vi "RTS Plot TCP Data.vi"(0 "Chamber 1 Socket":string[][](array[string]), 1 "Chamber 2 Socket":string[][](array[string]), 2 "Chamber 3 Socket":string[][](array[string]), 3 "Chamber 4 Socket":string[][](array[string]), 4 "Tree Selection in":T2, 5 "Error In":errorcluster, 9 "CSV Data in":T1 {"Station 1" format="%.6f"; "Station 2" format="%.6f"; "Station 3" format="%.6f"; "Station 4" format="%.6f"; "Station 5" format="%.6f"; "Station 6" format="%.6f"; "Station 7" format="%.6f"; "Station 8" format="%.6f"}) -> (10 "Chamber Data":string[][](array[string]), 13 "Full Item Names":string[](array[string]), 14 "Point File Name":string, 15 "CSV Data out":T1 {"Station 1" format="%.6f"; "Station 2" format="%.6f"; "Station 3" format="%.6f"; "Station 4" format="%.6f"; "Station 5" format="%.6f"; "Station 6" format="%.6f"; "Station 7" format="%.6f"; "Station 8" format="%.6f"}, 16 "Custom Titles":string[](array[string]), 17 "Listbox Data":string[][](array[string]), 18 "Tree Selection out":T2="Select Room/Stall", 19 "Error Out":errorcluster)   [LabVIEW 2020]
uses:
  Type Definitions/RTS TDMS Data.ctl
  Type Definitions/RTS Room Selector.ctl
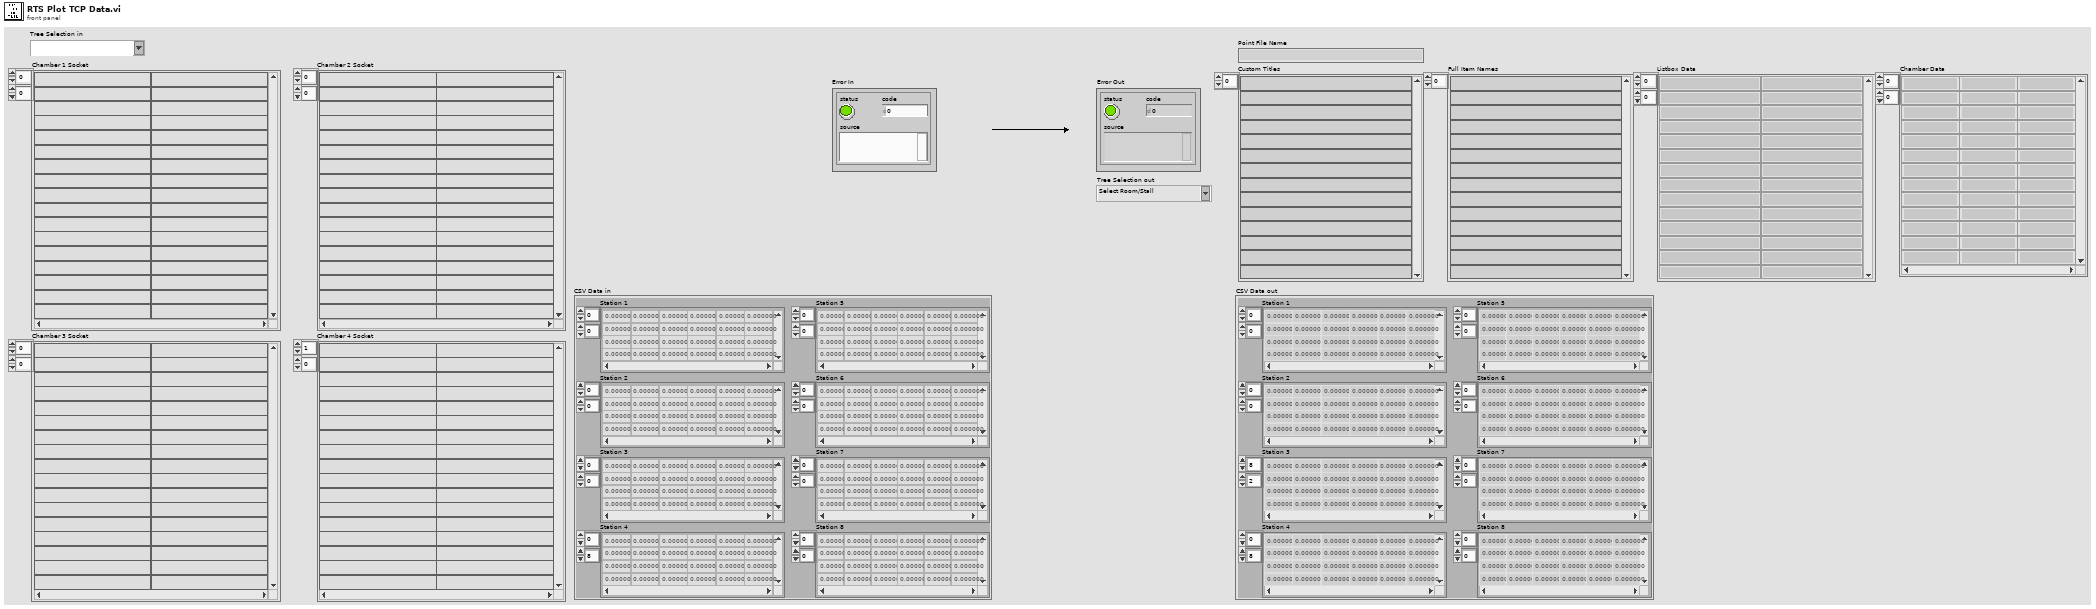
[diagram p1: front panel]
types:
  T1 = typedef "RTS TDMS Data.ctl" = cluster{"Station 1":dbl[][], "Station 2":dbl[][], "Station 3":dbl[][], "Station 4":dbl[][], "Station 5":dbl[][], "Station 6":dbl[][], "Station 7":dbl[][], "Station 8":dbl[][]}
  T2 = typedef "RTS Room Selector.ctl" = string
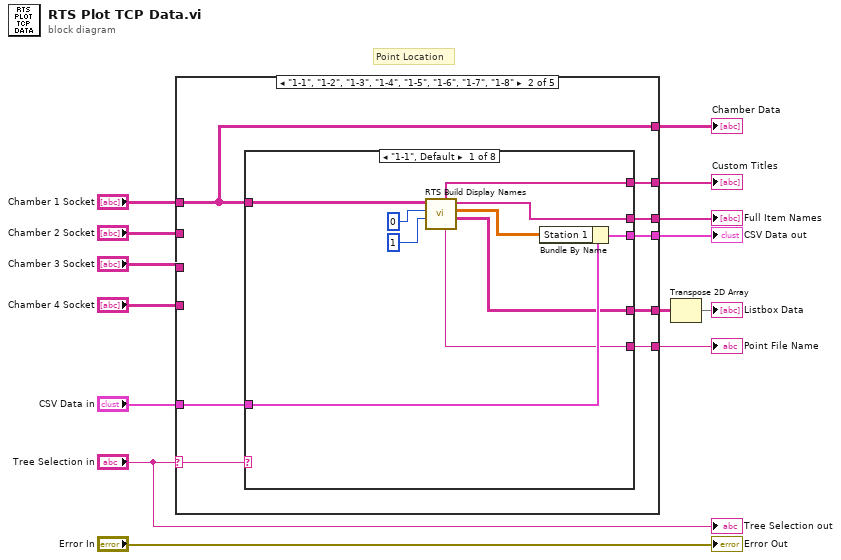
[diagram p0: block diagram]
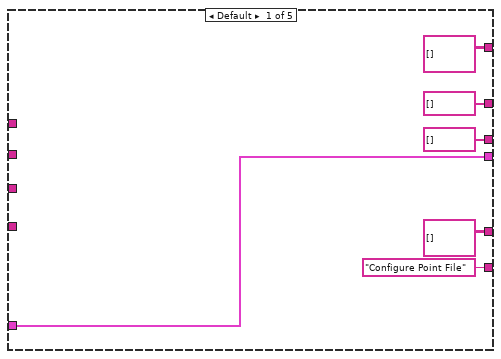
[diagram p2: hidden frame]
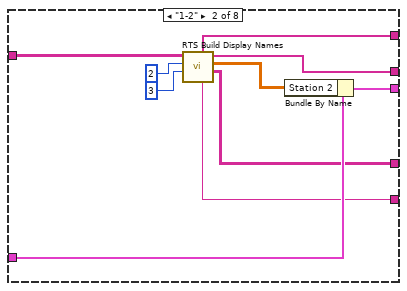
[diagram p3: hidden frame]
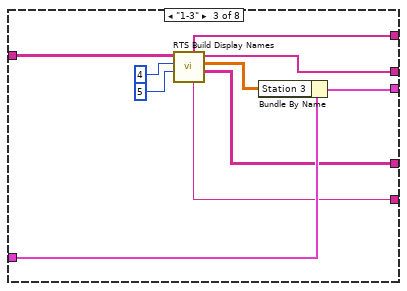
[diagram p4: hidden frame]
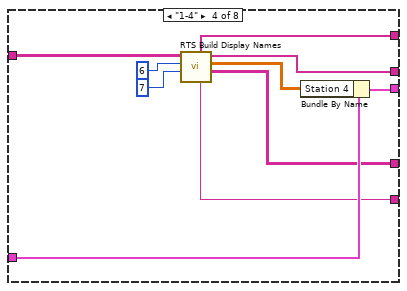
[diagram p5: hidden frame]
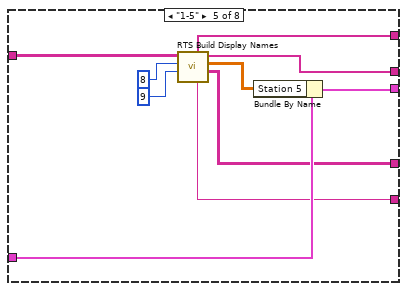
[diagram p6: hidden frame]
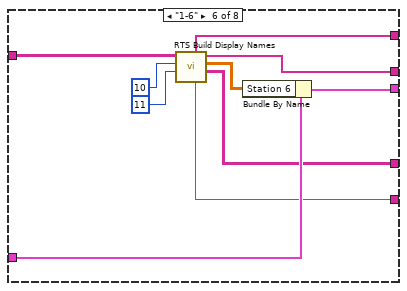
[diagram p7: hidden frame]
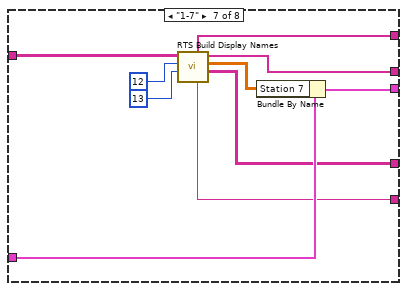
[diagram p8: hidden frame]
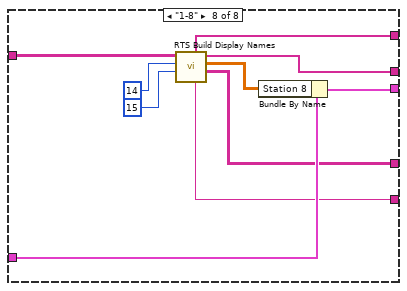
[diagram p9: hidden frame]
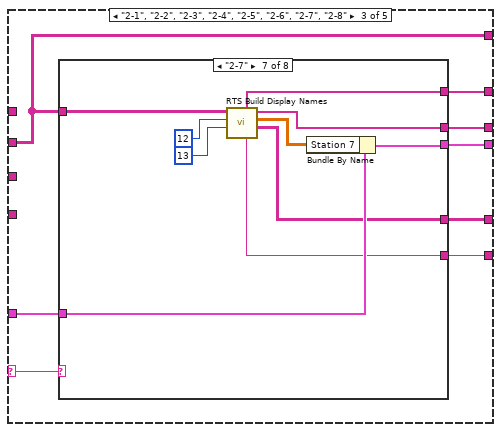
[diagram p10: hidden frame]
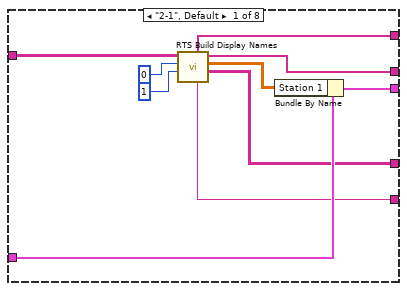
[diagram p11: hidden frame]
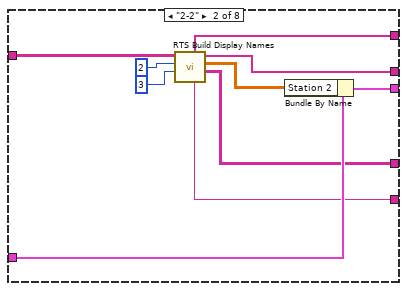
[diagram p12: hidden frame]
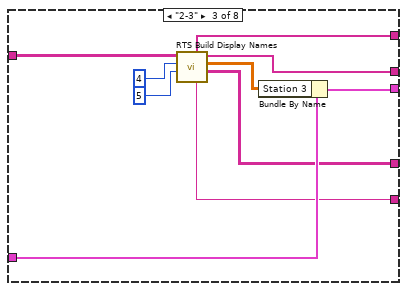
[diagram p13: hidden frame]
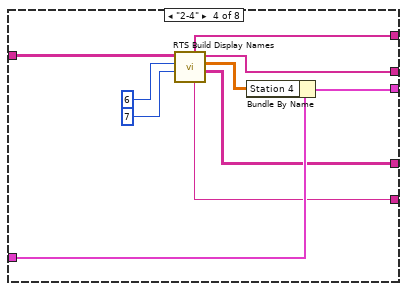
[diagram p14: hidden frame]
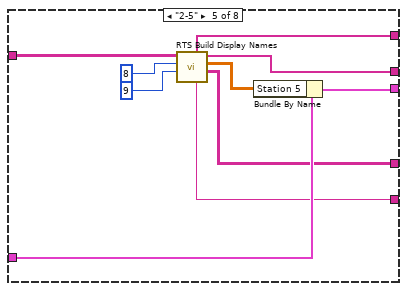
[diagram p15: hidden frame]
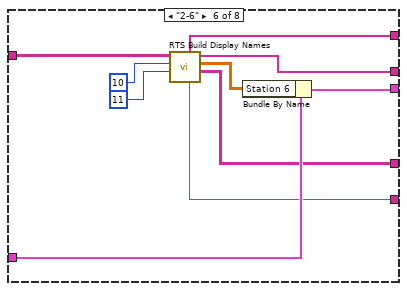
[diagram p16: hidden frame]
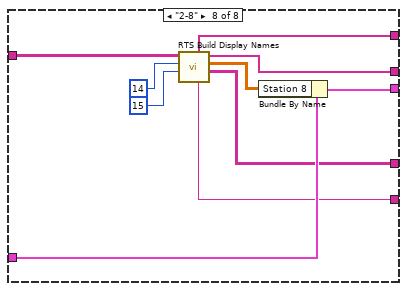
[diagram p17: hidden frame]
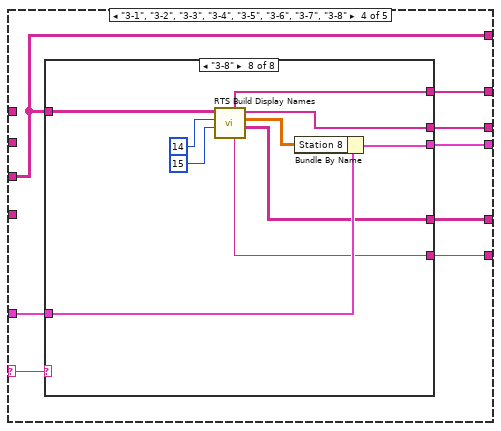
[diagram p18: hidden frame]
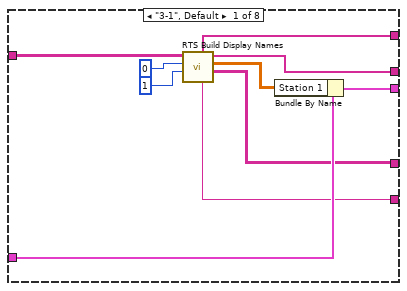
[diagram p19: hidden frame]
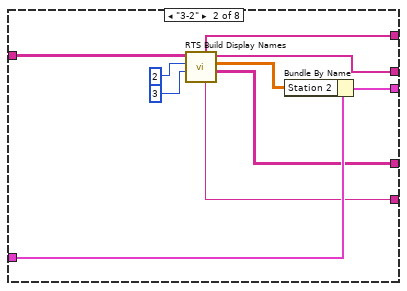
[diagram p20: hidden frame]
diagram:
  # "Point Location"
  n1 = case shown="\"1-1\", \"1-2\", \"1-3\", \"1-4\", \"1-5\", \"1-6\", \"1-7\", \"1-8\"" "Tree Selection in" {
    selector: "Tree Selection in" -> [_ w25 w113 w203 w291]
    tunnel: "Chamber 1 Socket" -> [_ w23 _ _ _]
    tunnel: "Chamber 2 Socket" -> [_ _ w111 _ _]
    tunnel: "Chamber 3 Socket" -> [_ _ _ w199 _]
    tunnel: "Chamber 4 Socket" -> [_ _ _ _ w287]
    tunnel: [string[] [] ("Chamber 4 Socket") w28 w114 w202 w290] -> w14
    tunnel: "CSV Data in" -> [w19 w27 w116 w204 w292]
    tunnel: [w19 w26 w115 w201 w289] -> w12
    tunnel: [string[][] [] w24 w112 w200 w288] -> w5
    tunnel: [string[][] [] ("Chamber 4 Socket") w23 w111 w199 w287] -> w3
    tunnel: [string[] [] ("Custom Titles") w22 w110 w198 w286] -> w2
    tunnel: ["Configure Point File" ("Point File Name") w21 w109 w197 w285] -> w1
    frame Default {
    }
    frame "1-1", "1-2", "1-3", "1-4", "1-5", "1-6", "1-7", "1-8" {
      n2 = case shown="\"1-1\", Default" w25 {
        tunnel: w23 -> [w38 w46 w56 w66 w76 w86 w96 w106]
        tunnel: [w32 w45 w53 w65 w75 w85 w95 w105] -> w28
        tunnel: w27 -> [w35 w48 w58 w68 w78 w88 w98 w108]
        tunnel: [w33 w47 w57 w67 w77 w87 w97 w107] -> w26
        tunnel: [w31 w43 w51 w63 w73 w83 w91 w103] -> w24
        tunnel: [w30 w40 w50 w60 w70 w80 w90 w100] -> w22
        tunnel: [w29 w39 w49 w59 w69 w79 w89 w99] -> w21
        frame "1-1", Default {
          n3 = call "RTS Build Display Names.vi"("Data Row"=1 ("index (row)"), "Name Row"=0 ("index (row)"), "Chamber 1 Socket in"=w38) -> ("Listbox Data"=w31:string[][], "DBL Plot Data"=w34:dbl[][], "Full Item Names"=w32:string[], "Point File Name"=w29:string, "Custom Titles"=w30:string[])  [unwired: 4 in]
          n4 = Bundle By Name(cluster=w35, "Station 1"=w34) -> (w33:T1)
        }
        frame "1-2" {
          n5 = call "RTS Build Display Names.vi"("Data Row"=3 ("index (row)"), "Name Row"=2 ("index (row)"), "Chamber 1 Socket in"=w46) -> ("Listbox Data"=w43:string[][], "DBL Plot Data"=w44:dbl[][], "Full Item Names"=w45:string[], "Point File Name"=w39:string, "Custom Titles"=w40:string[])  [unwired: 4 in]
          n6 = Bundle By Name(cluster=w48, "Station 2"=w44) -> (w47:T1)
        }
        frame "1-3" {
          n7 = call "RTS Build Display Names.vi"("Data Row"=5 ("index (row)"), "Name Row"=4 ("index (row)"), "Chamber 1 Socket in"=w56) -> ("Listbox Data"=w51:string[][], "DBL Plot Data"=w52:dbl[][], "Full Item Names"=w53:string[], "Point File Name"=w49:string, "Custom Titles"=w50:string[])  [unwired: 4 in]
          n8 = Bundle By Name(cluster=w58, "Station 3"=w52) -> (w57:T1)
        }
        frame "1-4" {
          n9 = call "RTS Build Display Names.vi"("Data Row"=7 ("index (row)"), "Name Row"=6 ("index (row)"), "Chamber 1 Socket in"=w66) -> ("Listbox Data"=w63:string[][], "DBL Plot Data"=w64:dbl[][], "Full Item Names"=w65:string[], "Point File Name"=w59:string, "Custom Titles"=w60:string[])  [unwired: 4 in]
          n10 = Bundle By Name(cluster=w68, "Station 4"=w64) -> (w67:T1)
        }
        frame "1-5" {
          n11 = call "RTS Build Display Names.vi"("Data Row"=9 ("index (row)"), "Name Row"=8 ("index (row)"), "Chamber 1 Socket in"=w76) -> ("Listbox Data"=w73:string[][], "DBL Plot Data"=w74:dbl[][], "Full Item Names"=w75:string[], "Point File Name"=w69:string, "Custom Titles"=w70:string[])  [unwired: 4 in]
          n12 = Bundle By Name(cluster=w78, "Station 5"=w74) -> (w77:T1)
        }
        frame "1-6" {
          n13 = call "RTS Build Display Names.vi"("Data Row"=11 ("index (row)"), "Name Row"=10 ("index (row)"), "Chamber 1 Socket in"=w86) -> ("Listbox Data"=w83:string[][], "DBL Plot Data"=w84:dbl[][], "Full Item Names"=w85:string[], "Point File Name"=w79:string, "Custom Titles"=w80:string[])  [unwired: 4 in]
          n14 = Bundle By Name(cluster=w88, "Station 6"=w84) -> (w87:T1)
        }
        frame "1-7" {
          n15 = call "RTS Build Display Names.vi"("Data Row"=13 ("index (row)"), "Name Row"=12 ("index (row)"), "Chamber 1 Socket in"=w96) -> ("Listbox Data"=w91:string[][], "DBL Plot Data"=w94:dbl[][], "Full Item Names"=w95:string[], "Point File Name"=w89:string, "Custom Titles"=w90:string[])  [unwired: 4 in]
          n16 = Bundle By Name(cluster=w98, "Station 7"=w94) -> (w97:T1)
        }
        frame "1-8" {
          n17 = call "RTS Build Display Names.vi"("Data Row"=15 ("index (row)"), "Name Row"=14 ("index (row)"), "Chamber 1 Socket in"=w106) -> ("Listbox Data"=w103:string[][], "DBL Plot Data"=w104:dbl[][], "Full Item Names"=w105:string[], "Point File Name"=w99:string, "Custom Titles"=w100:string[])  [unwired: 4 in]
          n18 = Bundle By Name(cluster=w108, "Station 8"=w104) -> (w107:T1)
        }
      }
    }
    frame "2-1", "2-2", "2-3", "2-4", "2-5", "2-6", "2-7", "2-8" {
      n19 = case shown="\"2-7\"" w113 {
        tunnel: w111 -> [w124 w134 w144 w154 w164 w174 w184 w194]
        tunnel: [w123 w133 w143 w153 w163 w173 w183 w193] -> w114
        tunnel: w116 -> [w126 w136 w146 w156 w166 w176 w186 w196]
        tunnel: [w125 w135 w145 w155 w165 w175 w185 w195] -> w115
        tunnel: [w121 w131 w141 w151 w161 w171 w181 w189] -> w112
        tunnel: [w118 w128 w138 w148 w158 w168 w178 w188] -> w110
        tunnel: [w117 w127 w137 w147 w157 w167 w177 w187] -> w109
        frame "2-1", Default {
          n20 = call "RTS Build Display Names.vi"("Data Row"=1 ("index (row)"), "Name Row"=0 ("index (row)"), "Chamber 1 Socket in"=w124) -> ("Listbox Data"=w121:string[][], "DBL Plot Data"=w122:dbl[][], "Full Item Names"=w123:string[], "Point File Name"=w117:string, "Custom Titles"=w118:string[])  [unwired: 4 in]
          n21 = Bundle By Name(cluster=w126, "Station 1"=w122) -> (w125:T1)
        }
        frame "2-2" {
          n22 = call "RTS Build Display Names.vi"("Data Row"=3 ("index (row)"), "Name Row"=2 ("index (row)"), "Chamber 1 Socket in"=w134) -> ("Listbox Data"=w131:string[][], "DBL Plot Data"=w132:dbl[][], "Full Item Names"=w133:string[], "Point File Name"=w127:string, "Custom Titles"=w128:string[])  [unwired: 4 in]
          n23 = Bundle By Name(cluster=w136, "Station 2"=w132) -> (w135:T1)
        }
        frame "2-3" {
          n24 = call "RTS Build Display Names.vi"("Data Row"=5 ("index (row)"), "Name Row"=4 ("index (row)"), "Chamber 1 Socket in"=w144) -> ("Listbox Data"=w141:string[][], "DBL Plot Data"=w142:dbl[][], "Full Item Names"=w143:string[], "Point File Name"=w137:string, "Custom Titles"=w138:string[])  [unwired: 4 in]
          n25 = Bundle By Name(cluster=w146, "Station 3"=w142) -> (w145:T1)
        }
        frame "2-4" {
          n26 = call "RTS Build Display Names.vi"("Data Row"=7 ("index (row)"), "Name Row"=6 ("index (row)"), "Chamber 1 Socket in"=w154) -> ("Listbox Data"=w151:string[][], "DBL Plot Data"=w152:dbl[][], "Full Item Names"=w153:string[], "Point File Name"=w147:string, "Custom Titles"=w148:string[])  [unwired: 4 in]
          n27 = Bundle By Name(cluster=w156, "Station 4"=w152) -> (w155:T1)
        }
        frame "2-5" {
          n28 = call "RTS Build Display Names.vi"("Data Row"=9 ("index (row)"), "Name Row"=8 ("index (row)"), "Chamber 1 Socket in"=w164) -> ("Listbox Data"=w161:string[][], "DBL Plot Data"=w162:dbl[][], "Full Item Names"=w163:string[], "Point File Name"=w157:string, "Custom Titles"=w158:string[])  [unwired: 4 in]
          n29 = Bundle By Name(cluster=w166, "Station 5"=w162) -> (w165:T1)
        }
        frame "2-6" {
          n30 = call "RTS Build Display Names.vi"("Data Row"=11 ("index (row)"), "Name Row"=10 ("index (row)"), "Chamber 1 Socket in"=w174) -> ("Listbox Data"=w171:string[][], "DBL Plot Data"=w172:dbl[][], "Full Item Names"=w173:string[], "Point File Name"=w167:string, "Custom Titles"=w168:string[])  [unwired: 4 in]
          n31 = Bundle By Name(cluster=w176, "Station 6"=w172) -> (w175:T1)
        }
        frame "2-7" {
          n32 = call "RTS Build Display Names.vi"("Data Row"=13 ("index (row)"), "Name Row"=12 ("index (row)"), "Chamber 1 Socket in"=w184) -> ("Listbox Data"=w181:string[][], "DBL Plot Data"=w182:dbl[][], "Full Item Names"=w183:string[], "Point File Name"=w177:string, "Custom Titles"=w178:string[])  [unwired: 4 in]
          n33 = Bundle By Name(cluster=w186, "Station 7"=w182) -> (w185:T1)
        }
        frame "2-8" {
          n34 = call "RTS Build Display Names.vi"("Data Row"=15 ("index (row)"), "Name Row"=14 ("index (row)"), "Chamber 1 Socket in"=w194) -> ("Listbox Data"=w189:string[][], "DBL Plot Data"=w190:dbl[][], "Full Item Names"=w193:string[], "Point File Name"=w187:string, "Custom Titles"=w188:string[])  [unwired: 4 in]
          n35 = Bundle By Name(cluster=w196, "Station 8"=w190) -> (w195:T1)
        }
      }
    }
    frame "3-1", "3-2", "3-3", "3-4", "3-5", "3-6", "3-7", "3-8" {
      n36 = case shown="\"3-8\"" w203 {
        tunnel: w199 -> [w212 w222 w232 w242 w252 w262 w272 w282]
        tunnel: [w207 w220 w228 w241 w251 w261 w271 w281] -> w202
        tunnel: w204 -> [w214 w224 w234 w244 w254 w264 w274 w284]
        tunnel: [w213 w223 w233 w243 w253 w263 w273 w283] -> w201
        tunnel: [w209 w218 w226 w239 w249 w259 w269 w279] -> w200
        tunnel: [w208 w221 w227 w236 w246 w256 w266 w276] -> w198
        tunnel: [w205 w215 w225 w235 w245 w255 w265 w275] -> w197
        frame "3-1", Default {
          n37 = call "RTS Build Display Names.vi"("Data Row"=1 ("index (row)"), "Name Row"=0 ("index (row)"), "Chamber 1 Socket in"=w212) -> ("Listbox Data"=w209:string[][], "DBL Plot Data"=w206:dbl[][], "Full Item Names"=w207:string[], "Point File Name"=w205:string, "Custom Titles"=w208:string[])  [unwired: 4 in]
          n38 = Bundle By Name(cluster=w214, "Station 1"=w206) -> (w213:T1)
        }
        frame "3-2" {
          n39 = call "RTS Build Display Names.vi"("Data Row"=3 ("index (row)"), "Name Row"=2 ("index (row)"), "Chamber 1 Socket in"=w222) -> ("Listbox Data"=w218:string[][], "DBL Plot Data"=w219:dbl[][], "Full Item Names"=w220:string[], "Point File Name"=w215:string, "Custom Titles"=w221:string[])  [unwired: 4 in]
          n40 = Bundle By Name(cluster=w224, "Station 2"=w219) -> (w223:T1)
        }
        frame "3-3" {
          n41 = call "RTS Build Display Names.vi"("Data Row"=5 ("index (row)"), "Name Row"=4 ("index (row)"), "Chamber 1 Socket in"=w232) -> ("Listbox Data"=w226:string[][], "DBL Plot Data"=w229:dbl[][], "Full Item Names"=w228:string[], "Point File Name"=w225:string, "Custom Titles"=w227:string[])  [unwired: 4 in]
          n42 = Bundle By Name(cluster=w234, "Station 3"=w229) -> (w233:T1)
        }
        frame "3-4" {
          n43 = call "RTS Build Display Names.vi"("Data Row"=7 ("index (row)"), "Name Row"=6 ("index (row)"), "Chamber 1 Socket in"=w242) -> ("Listbox Data"=w239:string[][], "DBL Plot Data"=w240:dbl[][], "Full Item Names"=w241:string[], "Point File Name"=w235:string, "Custom Titles"=w236:string[])  [unwired: 4 in]
          n44 = Bundle By Name(cluster=w244, "Station 4"=w240) -> (w243:T1)
        }
        frame "3-5" {
          n45 = call "RTS Build Display Names.vi"("Data Row"=9 ("index (row)"), "Name Row"=8 ("index (row)"), "Chamber 1 Socket in"=w252) -> ("Listbox Data"=w249:string[][], "DBL Plot Data"=w250:dbl[][], "Full Item Names"=w251:string[], "Point File Name"=w245:string, "Custom Titles"=w246:string[])  [unwired: 4 in]
          n46 = Bundle By Name(cluster=w254, "Station 5"=w250) -> (w253:T1)
        }
        frame "3-6" {
          n47 = call "RTS Build Display Names.vi"("Data Row"=11 ("index (row)"), "Name Row"=10 ("index (row)"), "Chamber 1 Socket in"=w262) -> ("Listbox Data"=w259:string[][], "DBL Plot Data"=w260:dbl[][], "Full Item Names"=w261:string[], "Point File Name"=w255:string, "Custom Titles"=w256:string[])  [unwired: 4 in]
          n48 = Bundle By Name(cluster=w264, "Station 6"=w260) -> (w263:T1)
        }
        frame "3-7" {
          n49 = call "RTS Build Display Names.vi"("Data Row"=13 ("index (row)"), "Name Row"=12 ("index (row)"), "Chamber 1 Socket in"=w272) -> ("Listbox Data"=w269:string[][], "DBL Plot Data"=w270:dbl[][], "Full Item Names"=w271:string[], "Point File Name"=w265:string, "Custom Titles"=w266:string[])  [unwired: 4 in]
          n50 = Bundle By Name(cluster=w274, "Station 7"=w270) -> (w273:T1)
        }
        frame "3-8" {
          n51 = call "RTS Build Display Names.vi"("Data Row"=15 ("index (row)"), "Name Row"=14 ("index (row)"), "Chamber 1 Socket in"=w282) -> ("Listbox Data"=w279:string[][], "DBL Plot Data"=w280:dbl[][], "Full Item Names"=w281:string[], "Point File Name"=w275:string, "Custom Titles"=w276:string[])  [unwired: 4 in]
          n52 = Bundle By Name(cluster=w284, "Station 8"=w280) -> (w283:T1)
        }
      }
    }
    frame "4-1", "4-2", "4-3", "4-4", "4-5", "4-6", "4-7", "4-8" {
      n53 = case shown="\"4-8\"" w291 {
        tunnel: w287 -> [w300 w310 w320 w330 w340 w350 w360 w370]
        tunnel: [w299 w309 w319 w329 w339 w349 w359 w369] -> w290
        tunnel: w292 -> [w302 w312 w322 w332 w342 w352 w362 w372]
        tunnel: [w301 w311 w321 w331 w341 w351 w361 w371] -> w289
        tunnel: [w297 w307 w317 w327 w337 w347 w357 w367] -> w288
        tunnel: [w294 w304 w314 w324 w334 w344 w354 w364] -> w286
        tunnel: [w293 w303 w313 w323 w333 w343 w353 w363] -> w285
        frame "4-1", Default {
          n54 = call "RTS Build Display Names.vi"("Data Row"=1 ("index (row)"), "Name Row"=0 ("index (row)"), "Chamber 1 Socket in"=w300) -> ("Listbox Data"=w297:string[][], "DBL Plot Data"=w298:dbl[][], "Full Item Names"=w299:string[], "Point File Name"=w293:string, "Custom Titles"=w294:string[])  [unwired: 4 in]
          n55 = Bundle By Name(cluster=w302, "Station 1"=w298) -> (w301:T1)
        }
        frame "4-2" {
          n56 = call "RTS Build Display Names.vi"("Data Row"=3 ("index (row)"), "Name Row"=2 ("index (row)"), "Chamber 1 Socket in"=w310) -> ("Listbox Data"=w307:string[][], "DBL Plot Data"=w308:dbl[][], "Full Item Names"=w309:string[], "Point File Name"=w303:string, "Custom Titles"=w304:string[])  [unwired: 4 in]
          n57 = Bundle By Name(cluster=w312, "Station 2"=w308) -> (w311:T1)
        }
        frame "4-3" {
          n58 = call "RTS Build Display Names.vi"("Data Row"=5 ("index (row)"), "Name Row"=4 ("index (row)"), "Chamber 1 Socket in"=w320) -> ("Listbox Data"=w317:string[][], "DBL Plot Data"=w318:dbl[][], "Full Item Names"=w319:string[], "Point File Name"=w313:string, "Custom Titles"=w314:string[])  [unwired: 4 in]
          n59 = Bundle By Name(cluster=w322, "Station 3"=w318) -> (w321:T1)
        }
        frame "4-4" {
          n60 = call "RTS Build Display Names.vi"("Data Row"=7 ("index (row)"), "Name Row"=6 ("index (row)"), "Chamber 1 Socket in"=w330) -> ("Listbox Data"=w327:string[][], "DBL Plot Data"=w328:dbl[][], "Full Item Names"=w329:string[], "Point File Name"=w323:string, "Custom Titles"=w324:string[])  [unwired: 4 in]
          n61 = Bundle By Name(cluster=w332, "Station 4"=w328) -> (w331:T1)
        }
        frame "4-5" {
          n62 = call "RTS Build Display Names.vi"("Data Row"=9 ("index (row)"), "Name Row"=8 ("index (row)"), "Chamber 1 Socket in"=w340) -> ("Listbox Data"=w337:string[][], "DBL Plot Data"=w338:dbl[][], "Full Item Names"=w339:string[], "Point File Name"=w333:string, "Custom Titles"=w334:string[])  [unwired: 4 in]
          n63 = Bundle By Name(cluster=w342, "Station 5"=w338) -> (w341:T1)
        }
        frame "4-6" {
          n64 = call "RTS Build Display Names.vi"("Data Row"=11 ("index (row)"), "Name Row"=10 ("index (row)"), "Chamber 1 Socket in"=w350) -> ("Listbox Data"=w347:string[][], "DBL Plot Data"=w348:dbl[][], "Full Item Names"=w349:string[], "Point File Name"=w343:string, "Custom Titles"=w344:string[])  [unwired: 4 in]
          n65 = Bundle By Name(cluster=w352, "Station 6"=w348) -> (w351:T1)
        }
        frame "4-7" {
          n66 = call "RTS Build Display Names.vi"("Data Row"=13 ("index (row)"), "Name Row"=12 ("index (row)"), "Chamber 1 Socket in"=w360) -> ("Listbox Data"=w357:string[][], "DBL Plot Data"=w358:dbl[][], "Full Item Names"=w359:string[], "Point File Name"=w353:string, "Custom Titles"=w354:string[])  [unwired: 4 in]
          n67 = Bundle By Name(cluster=w362, "Station 7"=w358) -> (w361:T1)
        }
        frame "4-8" {
          n68 = call "RTS Build Display Names.vi"("Data Row"=15 ("index (row)"), "Name Row"=14 ("index (row)"), "Chamber 1 Socket in"=w370) -> ("Listbox Data"=w367:string[][], "DBL Plot Data"=w368:dbl[][], "Full Item Names"=w369:string[], "Point File Name"=w363:string, "Custom Titles"=w364:string[])  [unwired: 4 in]
          n69 = Bundle By Name(cluster=w372, "Station 8"=w368) -> (w371:T1)
        }
      }
    }
  }
  "CSV Data out" <- w12
  "Full Item Names" <- w14
  "Chamber Data" <- w3
  "Custom Titles" <- w2
  "Point File Name" <- w1
  n70 = Transpose 2D Array(2D array=w5) -> (transposed array=→"Listbox Data":string[][])
  "Tree Selection out" <- "Tree Selection in"
  "Error Out" <- "Error In"
